vi "Index_Data.vi"() -> ()   [LabVIEW 2019]
uses:
  Retrieval_result.ctl
  Unrock_Data.ctl
  Cluster67.ctl
  <vilib>/addons/database/Connection.llb/DB Tools Open Connec (Path).vi
  <vilib>/addons/database/_DB Variant To Data/Database Variant To Data.xnode
  <vilib>/addons/database/NI_Database_API.lvlib
  TEST.lvclass
panel:
  in  "报表类型":bool=TRUE
  in  "机器名称（首填）":string
  in  "Retrieval_Results":T1[](array[typedef])
  in  "压头编号":string
  in  "机型":string
  in  "制造编号":string
  in  "index":bool
  in  "停止":bool
  # "序号"
  # "生产日期"
  # "机型"
  # "制造编号"
  # "压头编号"
  # "详细数据"
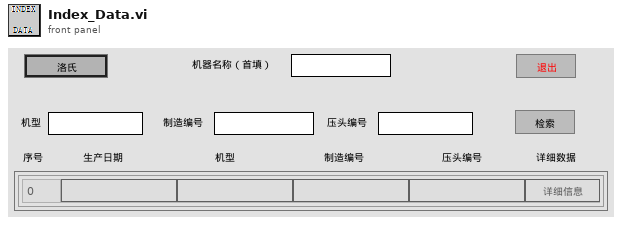
[diagram p1: front panel]
types:
  T1 = typedef "TEST.lvclass/Retrieval_result.ctl" = cluster{"序号":u16, "生产日期":string, "机型":string, "制造编号":string, "压头":string, "详细信息":bool}
  T2 = typedef "TEST.lvclass/Unrock_Data.ctl" = cluster{"MOD":string, "TSN":string, "Temp":string, "TEST1":sgl, "TEST2":sgl, "TEST3":sgl, "DEV":sgl, "INACC":sgl, "TEST1":sgl, "TEST2":sgl, "TEST3":sgl, "DEV":sgl, "INACC":sgl, "TEST1":sgl, "TEST2":sgl, "TEST3":sgl, "DEV":sgl, "INACC":sgl, "TEST1":sgl, "TEST2":sgl, "TEST3":sgl, "DEV":sgl, "INACC":sgl, "TEST1 5":sgl, "TEST2 5":sgl, "TEST3 5":sgl, "DEV 5":sgl, "INACC 5":sgl, "TEST1 4":sgl, "TEST2 4":sgl, "TEST3 4":sgl, "DEV 4":sgl, "INACC 4":sgl, "TEST1 3":sgl, "TEST2 3":sgl, "TEST3 3":sgl, "DEV 3":sgl, "INACC 3":sgl, "TEST1 2":sgl, "TEST2 2":sgl, "TEST3 2":sgl, "DEV 2":sgl, "INACC 2":sgl, "DIN":string, "HN":string, "HS":sgl, "TV1":sgl, "TV2":sgl, "TV3":sgl, "TV4":sgl, "TV5":sgl, "AVG":sgl, "HV":sgl, "REP":sgl, "HN":string, "HS":sgl, "TV1":sgl, "TV2":sgl, "TV3":sgl, "TV4":sgl, "TV5":sgl, "AVG":sgl, "HV":sgl, "REP":sgl, "HN":string, "HS":sgl, "TV1":sgl, "TV2":sgl, "TV3":sgl, "TV4":sgl, "TV5":sgl, "AVG":sgl, "HV":sgl, "REP":sgl, "HN":string, "HS":sgl, "TV1":sgl, "TV2":sgl, "TV3":sgl, "TV4":sgl, "TV5":sgl, "AVG":sgl, "HV":sgl, "REP":sgl, "HN":string, "HS":sgl, "TV1":sgl, "TV2":sgl, "TV3":sgl, "TV4":sgl, "TV5":sgl, "AVG":sgl, "HV":sgl, "REP":sgl, "NAM":string, "TDN":string, "PROD":string, "CALD":string, "REV":string}
  T3 = typedef "TEST.lvclass/Cluster67.ctl" = cluster{"MOD":string, "TSN":string, "Temp":string, "TEST1":sgl, "TEST2":sgl, "TEST3":sgl, "DEV":sgl, "INACC":sgl, "TEST1":sgl, "TEST2":sgl, "TEST3":sgl, "DEV":sgl, "INACC":sgl, "TEST1":sgl, "TEST2":sgl, "TEST3":sgl, "DEV":sgl, "INACC":sgl, "TEST1":sgl, "TEST2":sgl, "TEST3":sgl, "DEV":sgl, "INACC":sgl, "DIN":string, "HN":string, "HS":sgl, "TV1":sgl, "TV2":sgl, "TV3":sgl, "TV4":sgl, "TV5":sgl, "AVG":sgl, "HV":sgl, "REP":sgl, "HN":string, "HS":sgl, "TV1":sgl, "TV2":sgl, "TV3":sgl, "TV4":sgl, "TV5":sgl, "AVG":sgl, "HV":sgl, "REP":sgl, "HN":string, "HS":sgl, "TV1":sgl, "TV2":sgl, "TV3":sgl, "TV4":sgl, "TV5":sgl, "AVG":sgl, "HV":sgl, "REP":sgl, "HN":string, "HS":sgl, "TV1":sgl, "TV2":sgl, "TV3":sgl, "TV4":sgl, "TV5":sgl, "AVG":sgl, "HV":sgl, "REP":sgl, "HN":string, "HS":sgl, "TV1":sgl, "TV2":sgl, "TV3":sgl, "TV4":sgl, "TV5":sgl, "AVG":sgl, "HV":sgl, "REP":sgl, "NAM":string, "TDN":string, "PROD":string, "CALD":string, "REV":string}
  T4 = typedef "NI_Database_API.lvlib/Conn ObjectReference.ctl" = refnum<k1>
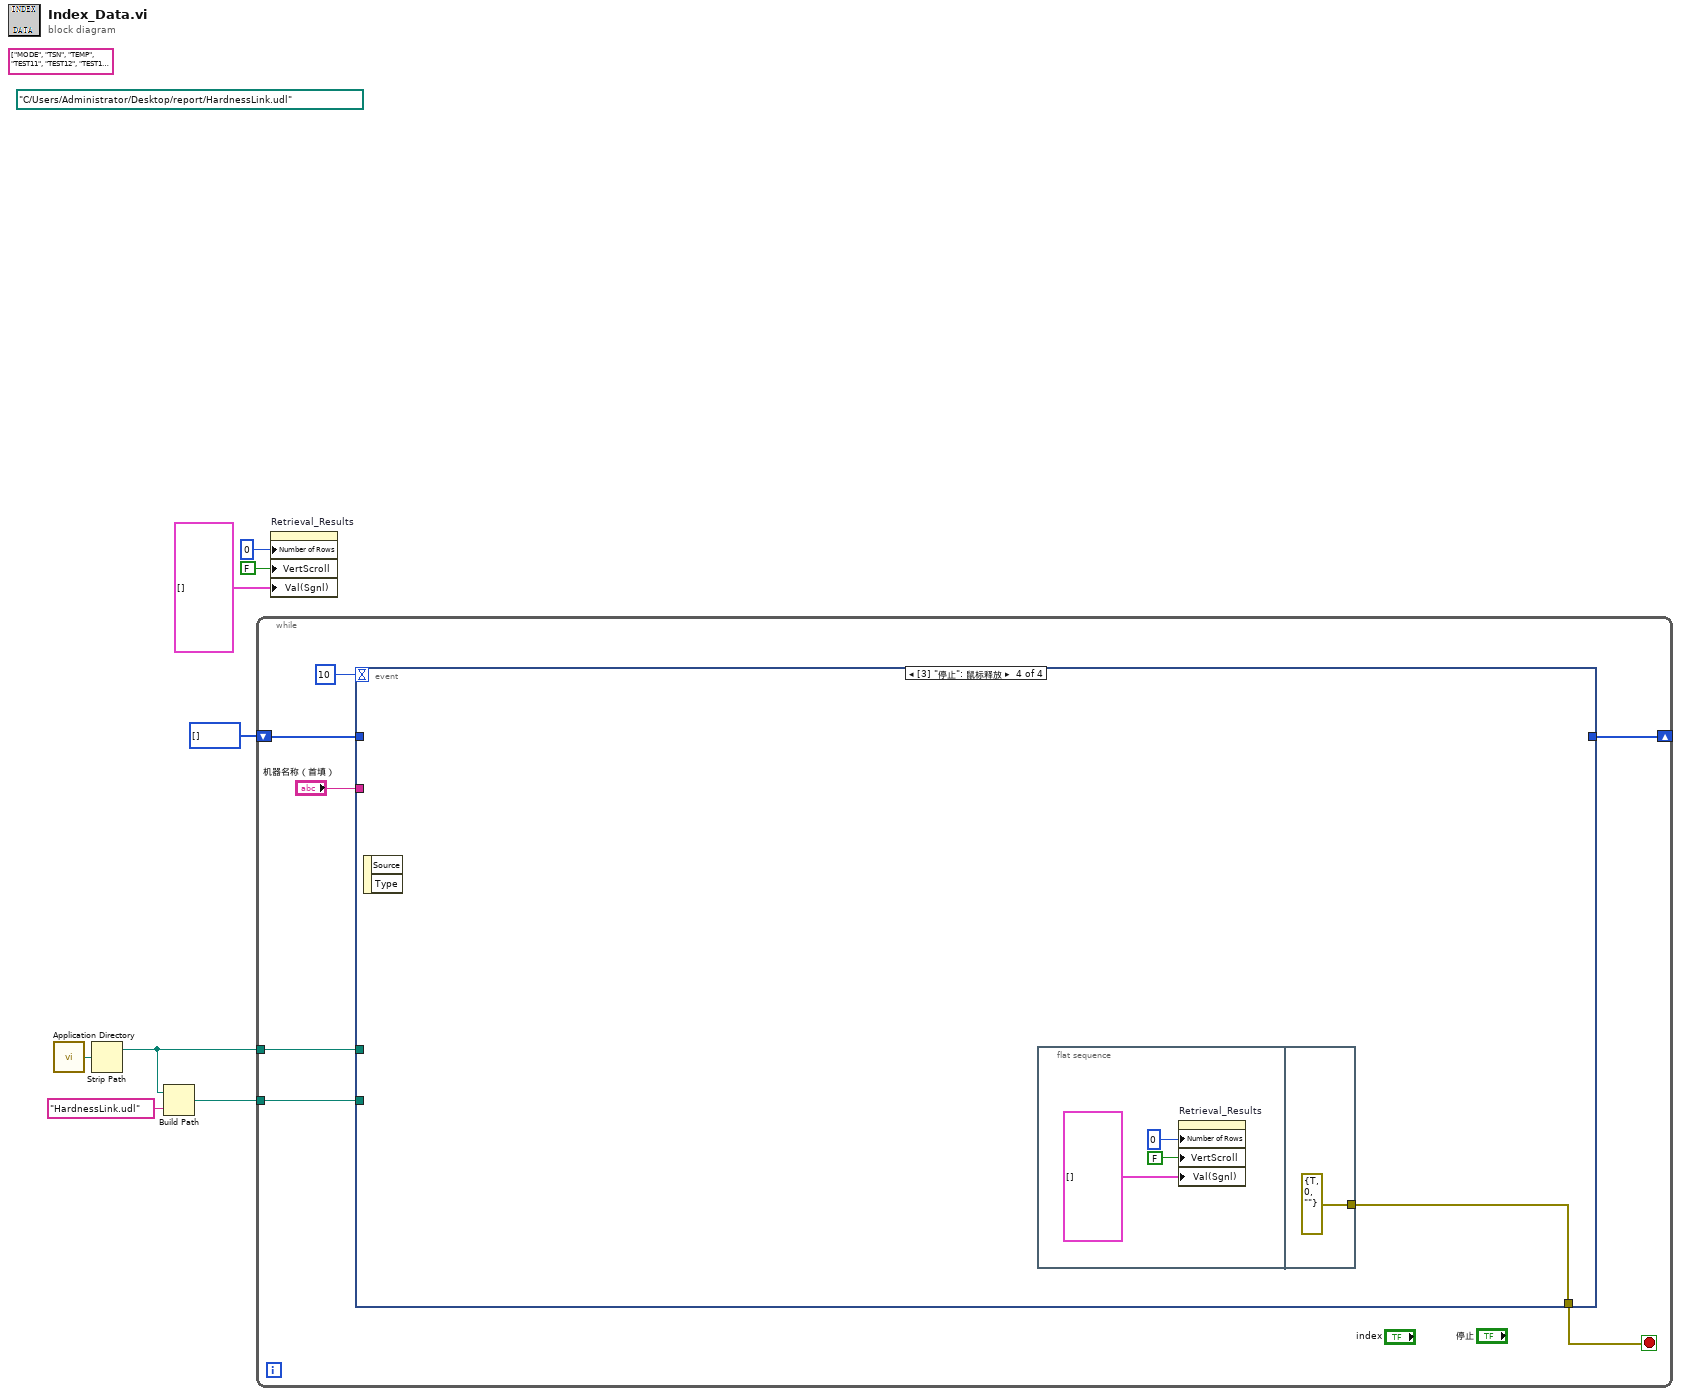
[diagram p0: block diagram]
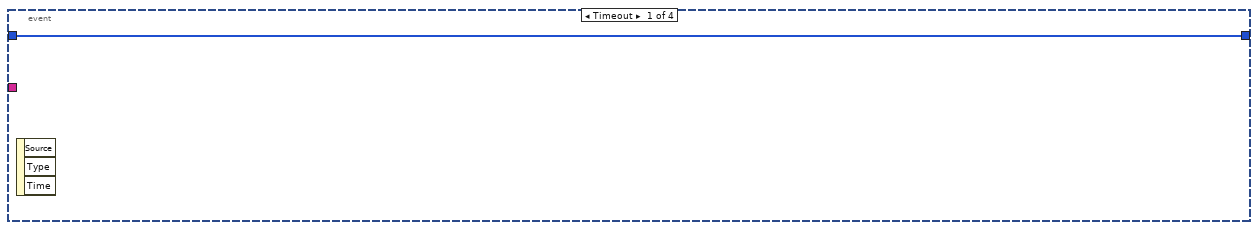
[diagram p2: hidden frame]
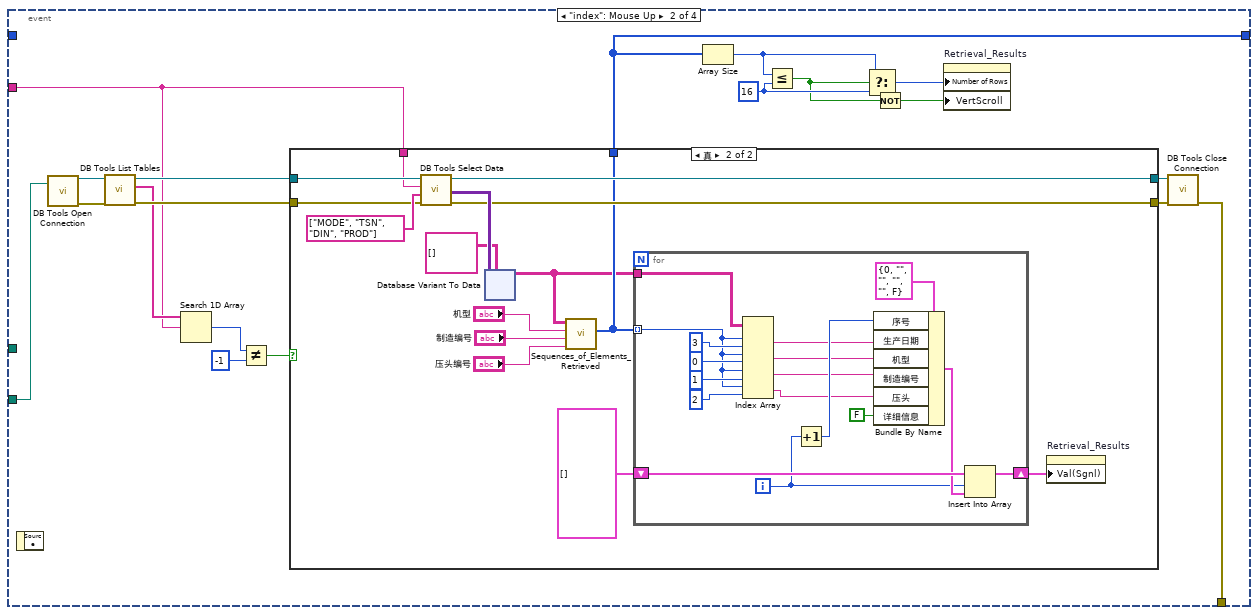
[diagram p3: hidden frame]
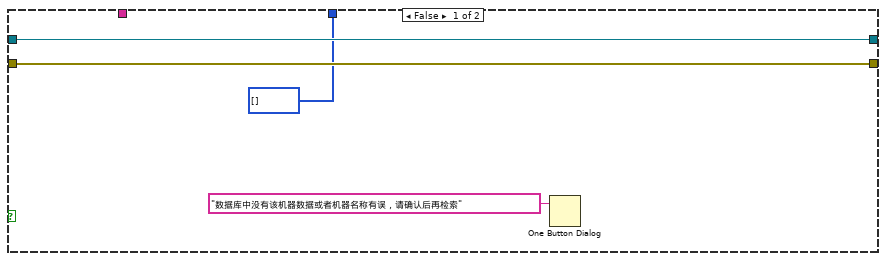
[diagram p4: hidden frame]
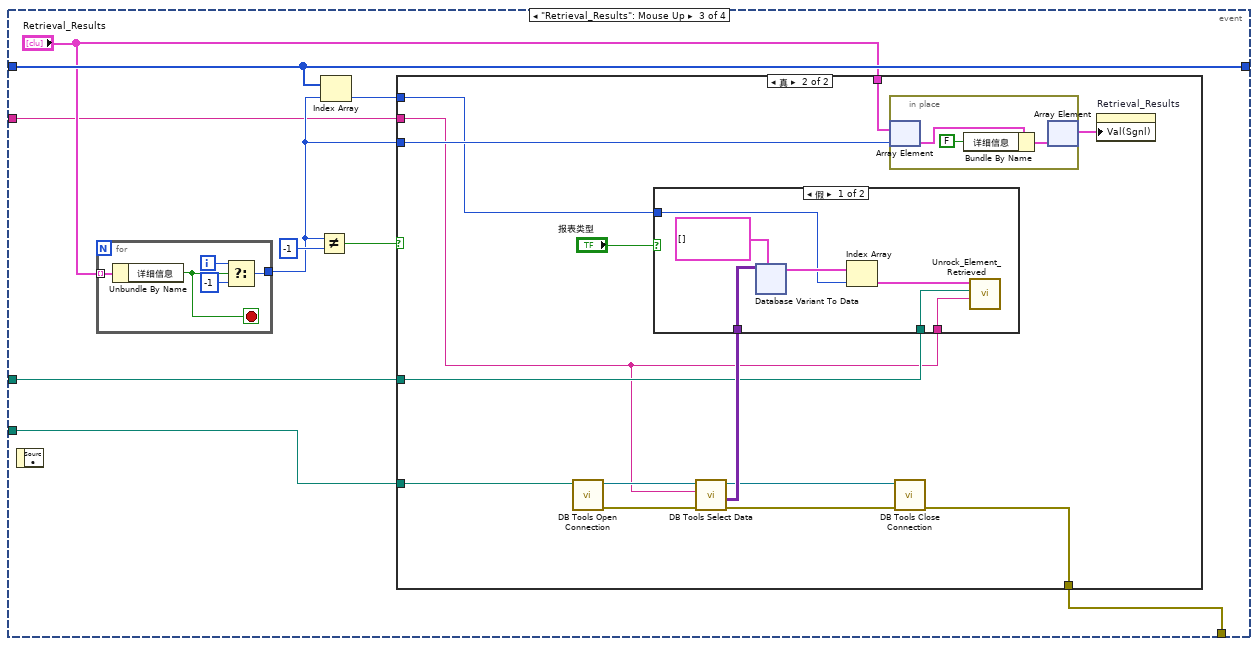
[diagram p5: hidden frame]
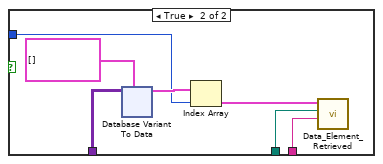
[diagram p7: hidden frame]
diagram:
  (unwired) string[] ["MODE", "TSN", "TEMP", "TEST11", "TEST12", "TEST13", "DEV1", "INACC1", "TEST21", "TEST22", "TEST23", "DEV2", "INACC2", "TEST31", "TEST32", "TEST33", "DEV3", "INACC3", "TEST41", "TEST42", "TEST43", "DEV4", "INACC4", "DIN", "HN1", "HS1", "TV11", "TV12", "TV13", "TV14", "TV15", "AVG1", "HV1", "REP1", "HN2", "HS2", "TV21", "TV22", "TV23", "TV24", "TV25", "AVG2", "HV2", "REP2", "HN3", "HS3", "TV31", "TV32", "TV33", "TV34", "TV35", "AVG3", "HV3", "REP3", "HN4", "HS4", "TV41", "TV42", "TV43", "TV44", "TV45", "AVG4", "HV4", "REP4", "HN5", "HS5", "TV51", "TV52", "TV53", "TV54", "TV55", "AVG5", "HV5", "REP5"] ("columns")
  (unwired) path "C:/Users/Administrator/Desktop/report/HardnessLink.udl" ("路径")
  n1 = call <vilib>:"Application Directory.vi"() -> ("Application Directory"=w4:path)
  n2 = Strip Path(path=w4) -> (stripped path=w3:path)  [unwired: 1 out]
  n3 = Build Path(base path=w3, name or relative path="HardnessLink.udl" ("名称或相对路径")) -> (appended path=w1:path)
  n4 = while {
    shift-right: [w14] -> _
    shift-left: i32[] [] -> [w13]
    tunnel: w3 -> [w10]
    tunnel: w1 -> [w9]
    stop <- w15 stop-if-true
    n5 = event shown="[3] \"停止\": 鼠标释放" {
      selector: _ -> [_ _ _ _]
      dyn-events: _ -> [_ _ _ _]
      timeout: 10 -> [_ _ _ _]
      tunnel: [_ w26 w118 w5700] -> w15
      tunnel: [w16 w30 w124 _] -> w14
      tunnel: w13 -> [w16 _ w124 _]
      tunnel: "机器名称（首填）" -> [_ w20 w119 _]
      tunnel: w10 -> [_ _ w117 _]
      tunnel: w9 -> [_ w25 w116 _]
      event Timeout {
        n6 = event-data() -> ()  [unwired: 1 in, 3 out]
      }
      event "index": Mouse Up {
        w35 = 16 ("y")
        n7 = event-data() -> ()  [unwired: 1 in, 1 out]
        n8 = call-poly <vilib>:"DB Tools Open Connection.vi"("connection information"=w25) -> ("error out"=w23:errorcluster, "connection reference"=w27:T4)  [unwired: 7 in]
        n9 = call <vilib>:"DB Tools List Tables.vi"("error in (no error)"=w23, "connection reference"=w27) -> ("error out"=w22:errorcluster, "tables"=w21:string[], "connection reference out"=w24:T4)  [unwired: 3 in]
        n10 = Search 1D Array(1D array=w21, element=w20) -> (index of element=w18:i32)  [unwired: 1 in]
        n11 = Not Equal?(x=w18, y=-1) -> (x != y?=w19:bool)
        n12 = case shown="真" w19 {
          tunnel: [w38 w50] -> w32
          tunnel: [w39 w49] -> w31
          tunnel: [i32[] [] w48] -> w30
          tunnel: w24 -> [w39 w42]
          tunnel: w22 -> [w38 w41]
          tunnel: w20 -> [_ w40]
          frame False {
            n13 = One Button Dialog(message="数据库中没有该机器数据或者机器名称有误，请确认后再检索" ("消息")) -> ()  [unwired: 1 in, 1 out]
          }
          frame True {
            n14 = call <vilib>:"DB Tools Select Data.vi"("error in (no error)"=w41, "columns"=string[] ["MODE", "TSN", "DIN", "PROD"], "table"=w40, "connection reference"=w42) -> ("error out"=w50:errorcluster, "data"=w53:variant[][], "connection reference out"=w49:T4)  [unwired: 2 in]
            n15 = xnode "Database Variant To Data"("database variant"=w53, "type"=string[][] []) -> ("data"=w43:string[][])  [unwired: 1 in, 1 out]
            n16 = call "Sequences_of_Elements_Retrieved.vi"("Element3"="压头编号", "Element2"="制造编号", "Element1"="机型", "Array_Retrieved"=w43) -> ("All_Data_Sequences"=w48:i32[])  [unwired: 7 in]
            n17 = for {
              tunnel: w48 -> [w60] mode=indexing
              shift-right: [w69] -> w47
              shift-left: T1[] [] -> [w68]
              tunnel: w43 -> [w55]
              i -> [w65]
              n18 = Index Array(array=w55, index (row) #1=w60, index (col) #1=3 ("禁用的索引 (列)"), index (row) #2=w60, index (col) #2=0 ("索引 (列)"), index (row) #3=w60, index (col) #3=1 ("索引 (列)"), index (row) #4=w60, index (col) #4=2 ("索引 (列)")) -> (element #1=w59:string, element #2=w58:string, element #3=w57:string, element #4=w56:string)
              n19 = Increment(x=w65) -> (x+1=w66:i32)
              n20 = Bundle By Name(cluster=T1 {"序号"=0, "生产日期"="", "机型"="", "制造编号"="", "压头"="", "详细信息"=FALSE} ("Retrieval_Result"), "序号"=w66, "生产日期"=w59, "机型"=w58, "制造编号"=w57, "压头"=w56, "详细信息"=FALSE) -> (w67:T1)
              n21 = Insert Into Array(array=w68, index=w65, new element=w67) -> (w69:T1[])
            }
            n22 = property on="Retrieval_Results" class="Arr (严格)"("Val(Sgnl)"=w47) -> ()  [unwired: 2 in, 2 out]
          }
        }
        n23 = Array Size(array=w30) -> (size(s)=w34:i32)
        n24 = Less Or Equal?(x=w34, y=w35) -> (x <= y?=w33:bool)
        n25 = Select(t=w34, s=w33, f=w35) -> (s? t:f=w29:i32)
        n26 = Not(x=w33) -> (.not. x?=w28:bool)
        n27 = property on="Retrieval_Results" class="Arr (严格)"("Number of Rows"=w29, "VertScroll"=w28) -> ()  [unwired: 2 in, 2 out]
        n28 = call <vilib>:"DB Tools Close Connection.vi"("error in (no error)"=w32, "connection reference"=w31) -> ("error out"=w26:errorcluster)  [unwired: 5 in]
      }
      event "Retrieval_Results": Mouse Up {
        n29 = event-data() -> ()  [unwired: 1 in, 1 out]
        n30 = for {
          tunnel: [w5699] -> w121
          tunnel: "Retrieval_Results" -> [w5695] mode=indexing
          i -> [w5697]
          stop <- w5698 stop-if-true
          n31 = Unbundle By Name(w5695) -> ("详细信息"=w5698:bool)
          n32 = Select(t=w5697, s=w5698, f=-1) -> (s? t:f=w5699:i32)
        }
        n33 = Not Equal?(x=w121, y=-1) -> (x != y?=w123:bool)
        n34 = Index Array(array=w124, index=w121) -> (element=w122:i32)
        n35 = case shown="真" w123 {
          tunnel: w122 -> [_ w132]
          tunnel: w121 -> [_ w139]
          tunnel: "Retrieval_Results" -> [_ w135]
          tunnel: w119 -> [_ w129]
          tunnel: [_ w133] -> w118
          tunnel: w117 -> [_ w131]
          tunnel: w116 -> [_ w130]
          frame False {
          }
          frame True {
            n36 = call-poly <vilib>:"DB Tools Open Connection.vi"("connection information"=w130) -> ("error out"=w137:errorcluster, "connection reference"=w138:T4)  [unwired: 7 in]
            n37 = call <vilib>:"DB Tools Select Data.vi"("error in (no error)"=w137, "table"=w129, "connection reference"=w138) -> ("error out"=w126:errorcluster, "data"=w136:variant[][], "connection reference out"=w127:T4)  [unwired: 3 in]
            n38 = case shown="假" "报表类型" {
              tunnel: w136 -> [w146 w3232]
              tunnel: w131 -> [w141 w3228]
              tunnel: w132 -> [w143 w3226]
              tunnel: w129 -> [w140 w3227]
              frame False {
                n39 = xnode "Database Variant To Data"("database variant"=w146, "type"=T2[] []) -> ("data"=w144:T2[])  [unwired: 1 in, 1 out]
                n40 = Index Array(array=w144, index=w143) -> (element=w142:T2)
                n41 = call "Unrock_Element_Retrieved.vi"("文件名"=w140, "路径"=w141, "Cluster67"=w142) -> ()  [unwired: 9 in]
              }
              frame True {
                n42 = xnode "Database Variant To Data"("database variant"=w3232, "type"=T3[] []) -> ("data"=w3230:T3[])  [unwired: 1 in, 1 out]
                n43 = Index Array(array=w3230, index=w3226) -> (element=w3229:T3)
                n44 = call "Data_Element_Retrieved.vi"("文件名"=w3227, "路径"=w3228, "Cluster67"=w3229) -> ()  [unwired: 9 in]
              }
            }
            n45 = in-place {
              n46 = in-place-array #1(w135, w139) -> (w5693:T1)
              n47 = Bundle By Name(cluster=w5693, "详细信息"=FALSE) -> (w5692:T1)
              n48 = in-place-array #1(w5692) -> (w134:T1[])  [unwired: 1 out]
            }
            n49 = call <vilib>:"DB Tools Close Connection.vi"("error in (no error)"=w126, "connection reference"=w127) -> ("error out"=w133:errorcluster)  [unwired: 5 in]
            n50 = property on="Retrieval_Results" class="Arr (严格)"("Val(Sgnl)"=w134) -> ()  [unwired: 2 in, 2 out]
          }
        }
      }
      event "停止": Mouse Up {
        n51 = event-data() -> ()  [unwired: 1 in, 2 out]
        n52 = flat-sequence {
          tunnel: [errorcluster {"status"=TRUE, "code"=0, "source"=""} ("error out")] -> w5700
          frame #0 {
            n53 = property on="Retrieval_Results" class="Arr (严格)"("Number of Rows"=0, "VertScroll"=FALSE, "Val(Sgnl)"=T1[] [] ("值(信号)")) -> ()  [unwired: 2 in, 2 out]
          }
          frame #1 {
          }
        }
      }
    }
  }
  n54 = property on="Retrieval_Results" class="Arr (严格)"("Number of Rows"=0, "VertScroll"=FALSE, "Val(Sgnl)"=T1[] [] ("值(信号)")) -> ()  [unwired: 2 in, 2 out]
